vi "Test Inf at FOR LOOP N.vi"() -> ()   [LabVIEW 2014]
uses:
  Analyze/Analyze Classes/Analyze Fluence/Analyze Fluence.lvclass
  Analyze/Analyze Parameter/Analyze Parameter Fluence/Analyze Parameter Fluence.lvclass
  Analyze/Analyze Classes/Analyze BaseClass/Analyze BaseClass/Analyze BaseClass.lvclass
panel:
  out "error out":errorcluster
  out "Numeric 2":i32
  in  "N":dbl=inf
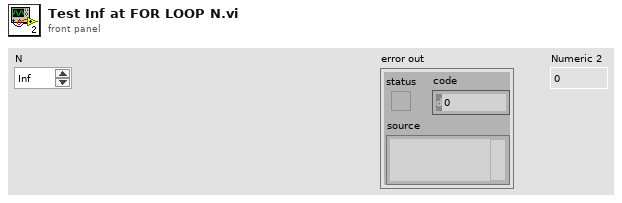
[diagram p1: front panel]
types:
  T1 = typedef "Image Type" = u32
  T2 = typedef "IMAQ Image.ctl" = refnum<image>
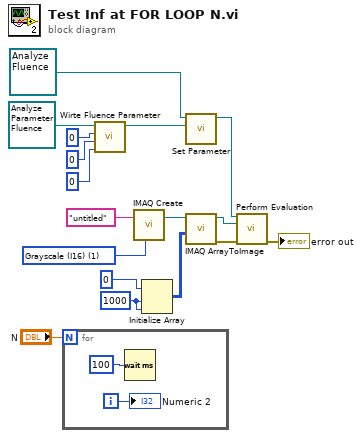
[diagram p0: block diagram]
diagram:
  w8 = T1 1 items=["Grayscale (U8)", "Grayscale (I16)", "Grayscale (SGL)", "Complex (CSG)", "RGB (U32)", "HSL (U32)", "RGB (U64)", "Grayscale (U16)"] ("Image Type")
  w15 = i16 1000
  n1 = for {
    N: "N" -> [_]
    i -> [w18]
    n2 = Wait (ms)(milliseconds to wait=u32 100) -> ()  [unwired: 1 out]
    "Numeric 2" <- w18
  }
  n3 = call "Wirte Fluence Parameter.vi"("#of Areas"=0, "#Overlays"=0, "Size of region (px)"=0, "Analyze Parameter Fluence in"=refnum<class "Analyze Parameter Fluence.lvclass"> refnum ("Analyze Parameter Fluence.lvclass")) -> ("Analyze Parameter Fluence out"=w4:refnum<class "Analyze Parameter Fluence.lvclass">)  [unwired: 7 in]
  n4 = call "IMAQ Create"("Image Name"="untitled", "Image Type"=w8) -> ("New Image"=w12:T2)  [unwired: 3 in, 1 out]
  n5 = Initialize Array(i16 0, w15, w15) -> (w13:i16[][])
  n6 = call-dynamic "Set Parameter.vi"("Analyze Parameter"=w4, "Analyze BaseClass in"=refnum<class "Analyze Fluence.lvclass"> refnum ("Analyze.lvlib:Analyze Fluence.lvclass")) -> ("Analyze BaseClass out"=w6:refnum<class "Analyze Fluence.lvclass">)  [unwired: 8 in, 1 out]
  n7 = call "IMAQ ArrayToImage"("Image Pixels (I16)"=w13, "Image"=w12) -> ("error out"=w11:errorcluster, "Image Out"=w10:T2)  [unwired: 8 in]
  n8 = call "Perform Evaluation.vi"("Analyze BaseClass in"=w6, "Image in"=w10, "error in (no error)"=w11) -> ("error out"=→"error out":errorcluster)  [unwired: 9 in, 3 out]
